vi "Termo_1.5__.vi"() -> ()   [LabVIEW 2015]
doc: "Программа мониторинга температуры"
uses:
  <vilib>/Utility/error.llb/DialogType.ctl
panel:
  in  "GraphLookB":bool
  out "Сутки":string
  out "счетчик":u32=4001
  in  "T min":u16=3 min=1 max=350
  in  "T max":u16=300 min=2 max=500
  in  "xScale -":bool
  in  "xScale +":bool
  out "мин.":string="20"
  out "TCP error source":string
  in  "порт":u16=4001
  in  "IP-адрес":string="10.10.10.2"
  out "Связь с прибором":bool
  in  "Disconnect":bool caption="Disconn"
  in  "Connect":bool
  out "3":bool
  out "1":bool
  out "2":bool
  out "Спаи":dbl format="%#_3g"
  out "K\n          Ом":dbl format="%#_5f"
  out "K\n          Ом 8":dbl format="%#_5f"
  out "K\n          Ом 7":dbl format="%#_5f"
  out "K\n          Ом 6":dbl format="%#_5f"
  out "Сол.":dbl format="%#_3g"
  out "Стр.":dbl format="%#_3g"
  out "Пер.":dbl format="%#_3g"
  out "4 2":bool
  in  "Запись в файл":bool
  out "сек.":string="0"
  out "часы":string="0"
  in  "Добавить время":dbl(ring)=300.0 items=["1 сек."=1.0, "10 сек."=10.0, "1 мин."=60.0, "5 мин."=300.0, "10 мин."=600.0, "1 час"=3600.0, ""=0.0]
  in  "stop":bool
  out "con err":bool caption="Connect"
  out "Graphs":dynamicdata(graph)
  out "read_error_indicator":bool
  out "refnum out":refnum<file>
  in  "flag1":bool caption="Disconn"
  out "x+1":dbl
  out "connection ID":refnum<k5>
  out "Расположение файла":path
  # "R [Ом]"
  # "T [K] [K]"
  # "Стр."
  # "Спаи"
  # "Пер."
  # "Сол."
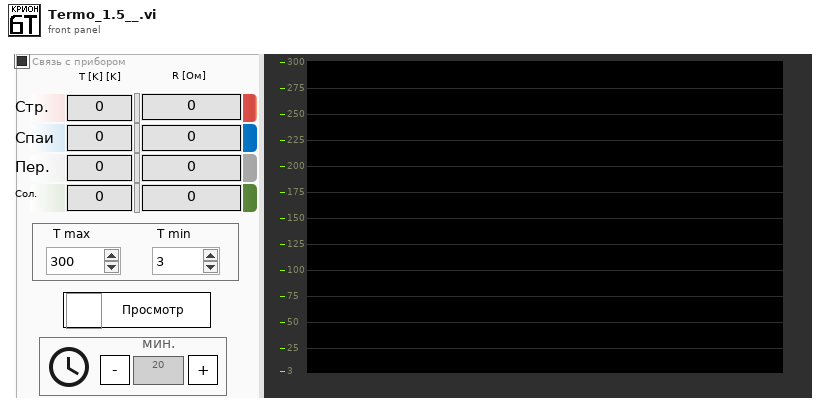
[diagram p1: front panel]
types:
  T1 = typedef "LVDateTimeRec.ctl" = cluster{"fractional second":dbl, "second":i32, "minute":i32, "hour":i32, "day of month":i32, "month":i32, "year":i32, "day of week":i32, "day of year":i32, "DST":i32}
  T2 = enum16{"Standard", "Buffered", "CRLF", "Immediate"}
  T3 = cluster{"y":ext, "y":ext, "y":ext, "y":ext, "y":ext, "y":ext, "y":ext}
  T4 = typedef "DialogType.ctl" = u16
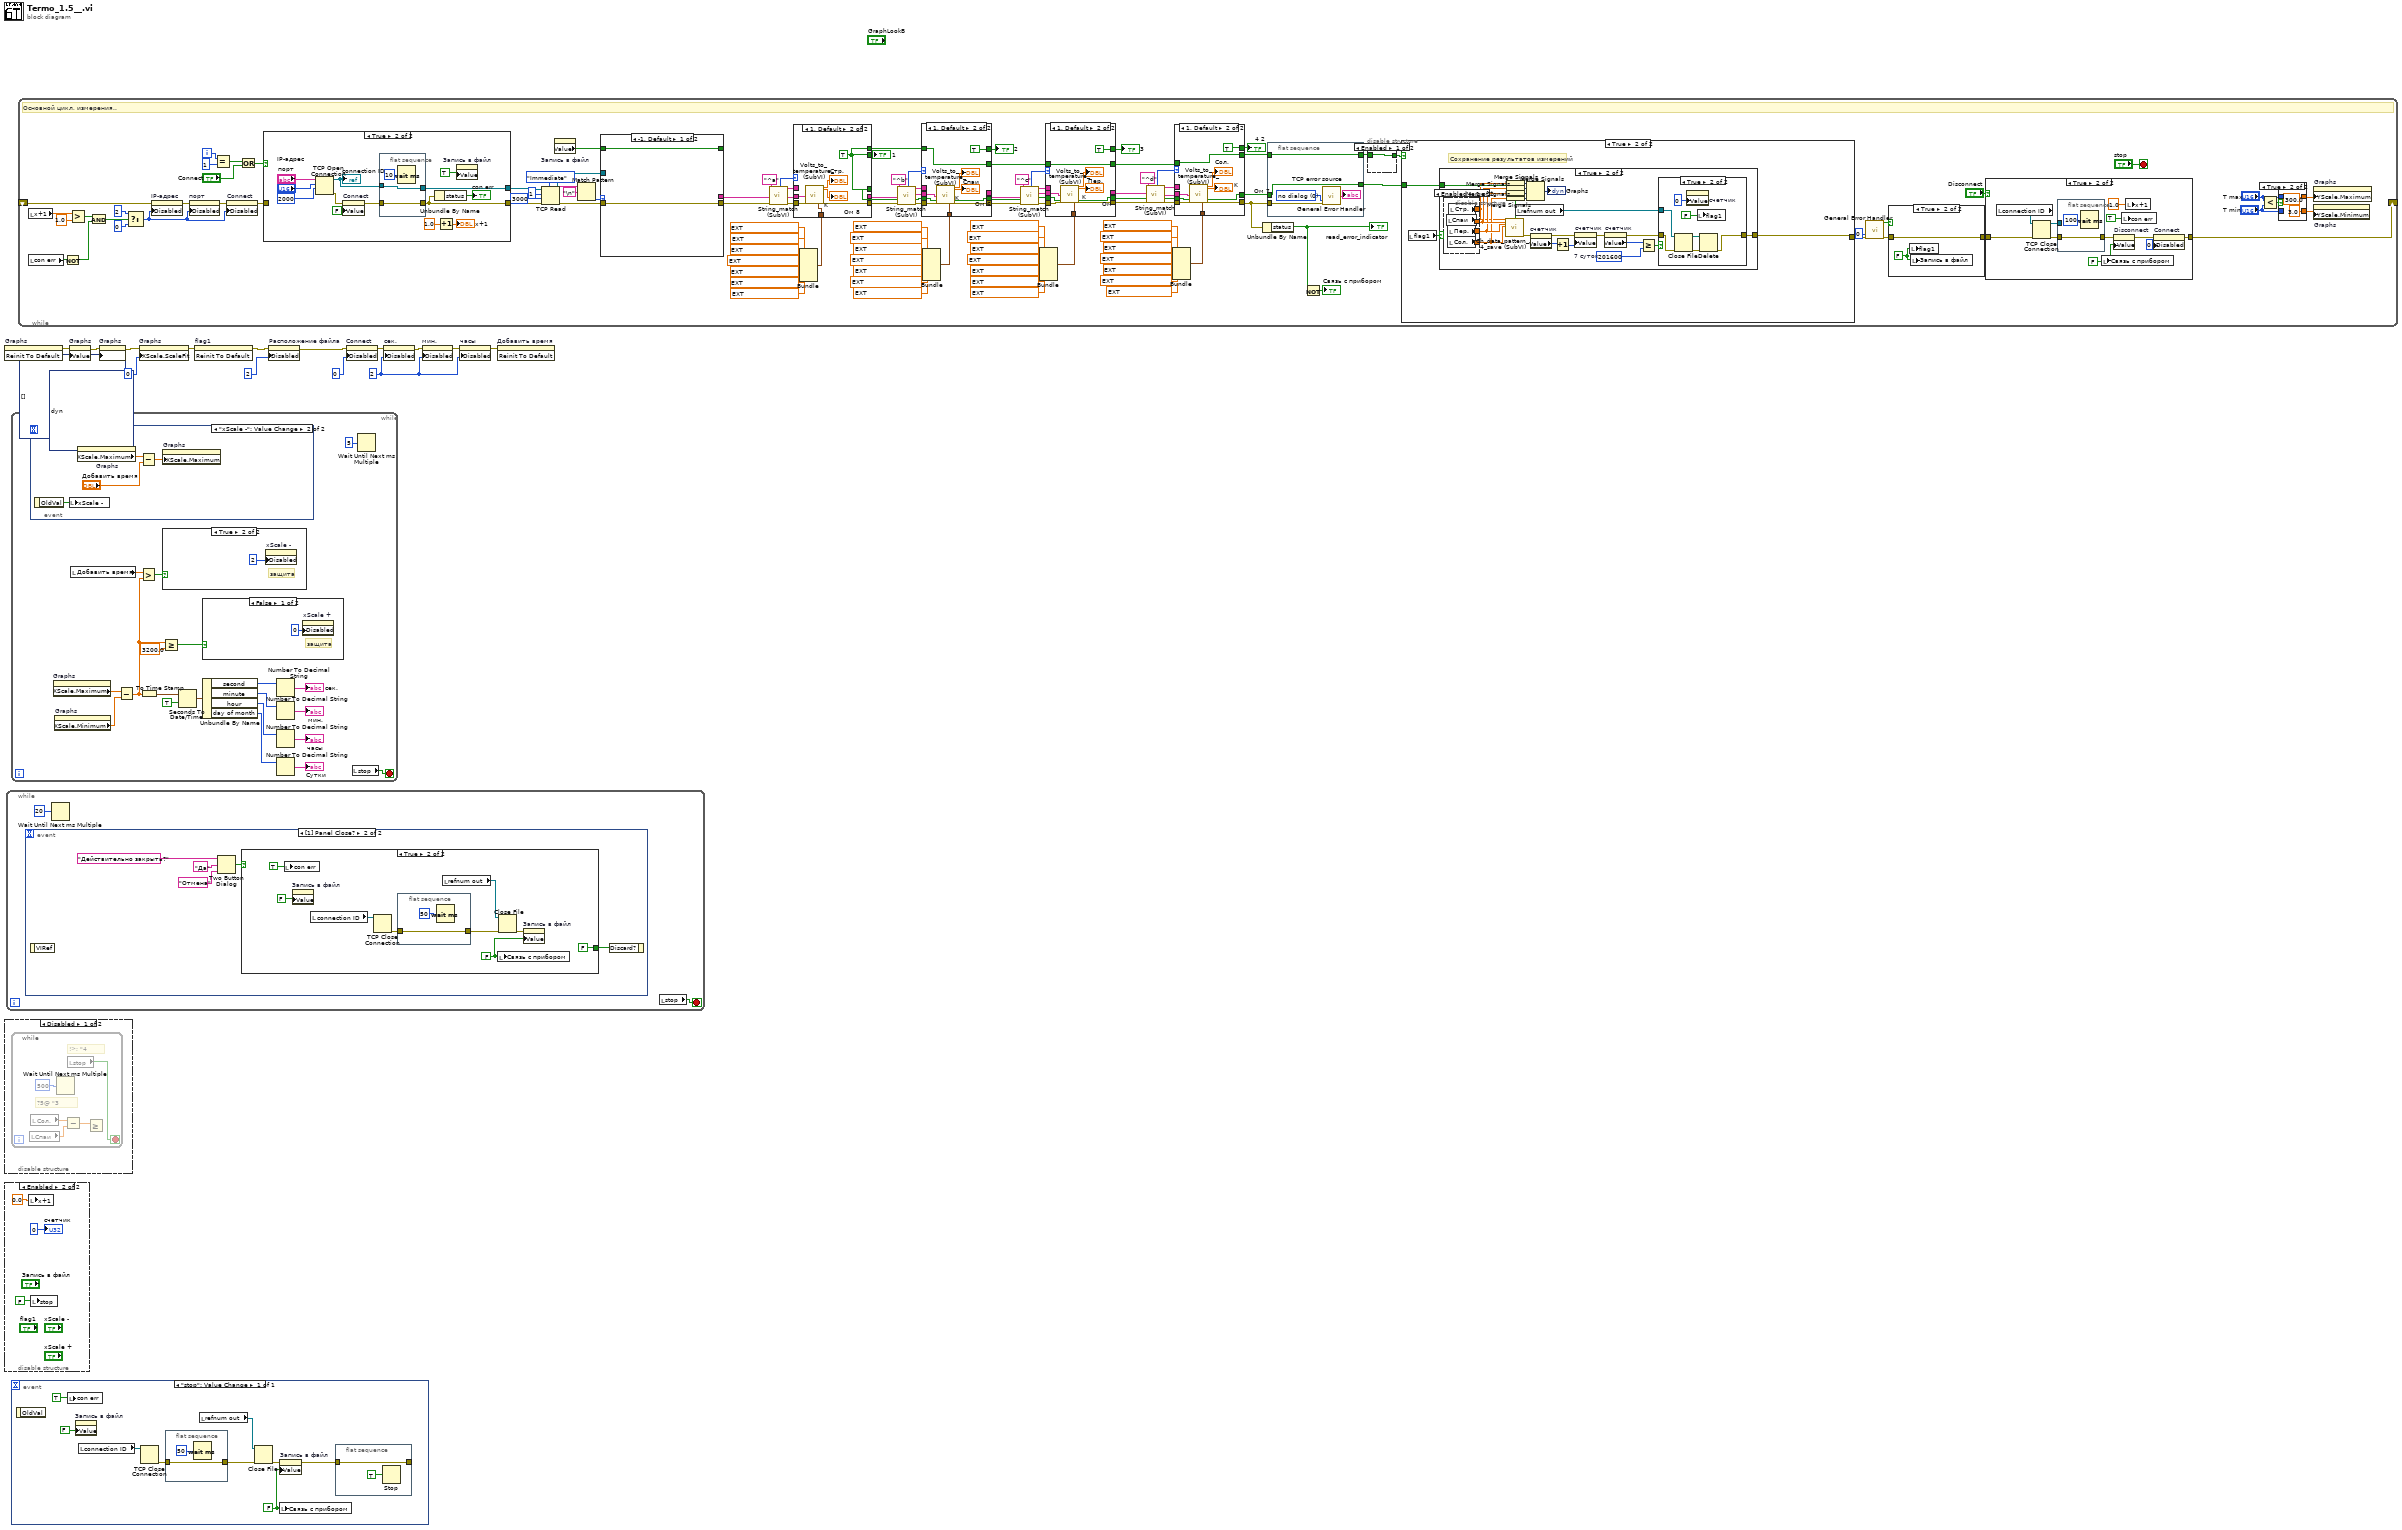
[diagram p0: block diagram]
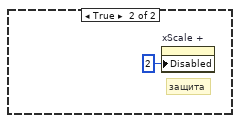
[diagram p2: hidden frame]
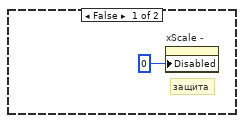
[diagram p3: hidden frame]
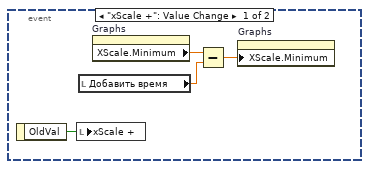
[diagram p4: hidden frame]
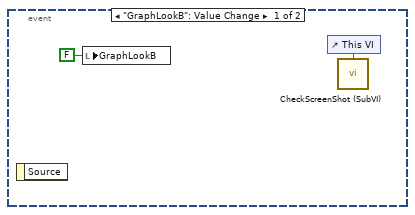
[diagram p7: hidden frame]
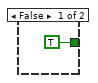
[diagram p8: hidden frame]
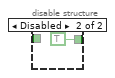
[diagram p9: hidden frame]
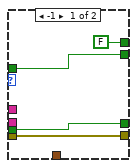
[diagram p11: hidden frame]
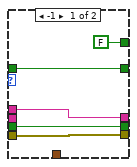
[diagram p12: hidden frame]
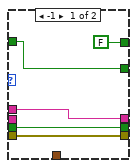
[diagram p13: hidden frame]
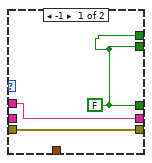
[diagram p14: hidden frame]
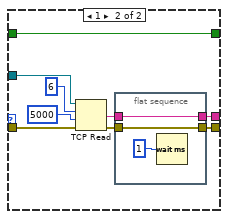
[diagram p15: hidden frame]
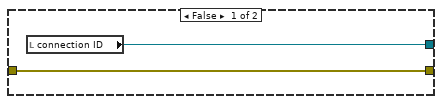
[diagram p16: hidden frame]
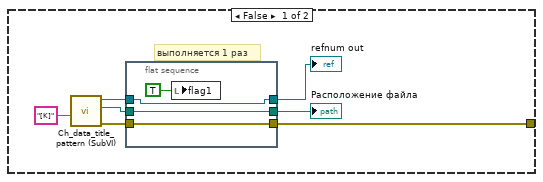
[diagram p19: hidden frame]
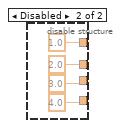
[diagram p20: hidden frame]
diagram:
  w15 = u8 2 ("Disabled")
  n1 = invoke on="Graphs" class="WFChart (strict)" method="Reinit To Default"() -> (error out=w7:errorcluster)  [unwired: 3 in, 2 out]
  n2 = disable-structure shown="Disabled" {
    frame Disabled {
      n3 = while {
        stop <- w23 stop-if-true
        # "!>; \"4"
        # "?5@ \"3"
        n4 = local read "Спаи"() -> (w19:dbl)
        n5 = local read "Сол."() -> (w20:dbl)
        n6 = Wait Until Next ms Multiple(millisecond multiple=u32 500) -> ()  [unwired: 1 out]
        n7 = Subtract(x=w20, y=w19) -> (x-y=w17:dbl)
        n8 = local read "stop"() -> (w23:bool)
        n9 = Greater Or Equal?(x=w17) -> (y=w18:dbl, x >= y?=w21:bool)
      }
    }
    frame Enabled {
    }
  }
  n10 = disable-structure shown="Enabled" {
    frame Disabled {
    }
    frame Enabled {
      n11 = local write "x+1"(0.0 ("x+1")) -> ()
      n12 = local write "stop"(FALSE ("Boolean")) -> ()
      "счетчик" <- u32 0 ("счетчик")
    }
  }
  n13 = while {
    stop <- w27 stop-if-true
    n14 = event shown="[1] Panel Close?" {
      selector: _ -> [_ _]
      dyn-events: _ -> [_ _]
      timeout: _ -> [_ _]
      event "GraphLookB": Value Change {
        n15 = event-data() -> ()  [unwired: 2 out]
        n16 = local write "GraphLookB"(FALSE ("Снимок")) -> ()
        n17 = control-ref of="This VI"() -> (w29:refnum<vi>)
        n18 = call "CheckScreenShot (SubVI).vi"("VI reference"=w29) -> ()  [unwired: 15 in]
      }
      event Panel Close? {
        n19 = event-data() -> ()  [unwired: 2 out]
        n20 = Two Button Dialog(message="Действительно закрыть?", 1:"Отмена" ("T button name (\"OK\")"), 2:"Да" ("T button name (\"OK\")")) -> (T button?=w35:bool)
        n21 = case shown="True" w35 {
          tunnel: [TRUE ("Discard?") FALSE ("Discard?")] -> w31
          frame False {
          }
          frame True {
            w42 = FALSE ("Запись в файл")
            n22 = local write "con err"(TRUE ("Tool Bar:Visible")) -> ()
            n23 = property on="Запись в файл" class="Bool (strict)"("Value"=FALSE ("Запись в файл")) -> ()  [unwired: 2 in, 2 out]
            n24 = local read "connection ID"() -> (w38:refnum<k5>)
            n25 = TCP Close Connection(connection ID=w38) -> (error out=w45:errorcluster)  [unwired: 1 in, 2 out]
            n26 = flat-sequence {
              tunnel: [w46] -> w44
              tunnel: w45 -> [w46]
              frame #0 {
                n27 = Wait (ms)(milliseconds to wait=u32 50) -> ()  [unwired: 1 out]
              }
            }
            n28 = local read "refnum out"() -> (w40:refnum<file>)
            n29 = local write "Связь с прибором"(w42) -> ()
            n30 = Close File(refnum=w40, error in=w44) -> (error out=w39:errorcluster)  [unwired: 1 out]
            n31 = property on="Запись в файл" class="Bool (strict)"(error in=w39, "Value"=w42) -> ()  [unwired: 1 in, 2 out]
          }
        }
        n32 = event-data("Discard?"=w31) -> ()  [unwired: 1 in, 1 out]
      }
    }
    n33 = Wait Until Next ms Multiple(millisecond multiple=u32 20) -> ()  [unwired: 1 out]
    n34 = local read "stop"() -> (w27:bool)
  }
  n35 = while {
    stop <- w67 stop-if-true
    n36 = event shown="[1] \"xScale -\": Value Change" {
      selector: _ -> [_ _]
      dyn-events: _ -> [_ _]
      timeout: _ -> [_ _]
      event "xScale +": Value Change {
        n37 = event-data() -> ("OldVal"=w72:bool)  [unwired: 1 in]
        n38 = local write "xScale +"(w72) -> ()
        n39 = local read "Добавить время"() -> (w75:dbl)
        n40 = property on="Graphs" class="WFChart (strict)"() -> ("XScale.Minimum"=w74:dbl)  [unwired: 2 in, 2 out]
        n41 = Subtract(x=w74, y=w75) -> (x-y=w73:dbl)
        n42 = property on="Graphs" class="WFChart (strict)"("XScale.Minimum"=w73) -> ()  [unwired: 2 in, 2 out]
      }
      event "xScale -": Value Change {
        n43 = event-data() -> ("OldVal"=w76:bool)  [unwired: 1 in]
        n44 = local write "xScale -"(w76) -> ()
        n45 = property on="Graphs" class="WFChart (strict)"() -> ("XScale.Maximum"=w78:dbl)  [unwired: 2 in, 2 out]
        n46 = Subtract(x=w78, y="Добавить время") -> (x-y=w77:dbl)
        n47 = property on="Graphs" class="WFChart (strict)"("XScale.Maximum"=w77) -> ()  [unwired: 2 in, 2 out]
      }
    }
    n48 = property on="Graphs" class="WFChart (strict)"() -> ("XScale.Maximum"=w66:dbl)  [unwired: 2 in, 2 out]
    n49 = property on="Graphs" class="WFChart (strict)"() -> ("XScale.Minimum"=w65:dbl)  [unwired: 2 in, 2 out]
    n50 = local read "Добавить время"() -> (w63:dbl)
    n51 = Subtract(x=w66, y=w65) -> (x-y=w51:dbl)
    n52 = Greater?(x=w63, y=w51) -> (0:w64:bool)
    n53 = To Time Stamp(1:w51) -> (0:w61:timestamp)
    n54 = Greater Or Equal?(x=w51, y=3200.0) -> (x >= y?=w49:bool)
    n55 = case shown="True" w64 {
      frame False {
        # "защита"
        n56 = property on="xScale -" class="Bool (strict)"("Disabled"=u8 0) -> ()  [unwired: 2 in, 2 out]
      }
      frame True {
        # "защита"
        n57 = property on="xScale -" class="Bool (strict)"("Disabled"=u8 2) -> ()  [unwired: 2 in, 2 out]
      }
    }
    n58 = Seconds To Date/Time(time stamp (now)=w61, to UTC (F)=TRUE) -> (date time rec=w60:T1)
    n59 = case shown="False" w49 {
      frame False {
        # "защита"
        n60 = property on="xScale +" class="Bool (strict)"("Disabled"=u8 0) -> ()  [unwired: 2 in, 2 out]
      }
      frame True {
        # "защита"
        n61 = property on="xScale +" class="Bool (strict)"("Disabled"=u8 2) -> ()  [unwired: 2 in, 2 out]
      }
    }
    n62 = Unbundle By Name(w60) -> ("second"=w59:i32, "minute"=w58:i32, "hour"=w57:i32, "day of month"=w56:i32)
    n63 = Number To Decimal String(number=w59) -> (decimal integer string=→"сек.":string)  [unwired: 1 out]
    n64 = Number To Decimal String(number=w58) -> (decimal integer string=→"мин.":string)  [unwired: 1 out]
    n65 = Number To Decimal String(number=w57) -> (decimal integer string=→"часы":string)  [unwired: 1 out]
    n66 = Number To Decimal String(number=w56) -> (decimal integer string=→"Сутки":string)  [unwired: 1 out]
    n67 = local read "stop"() -> (w67:bool)
    n68 = Wait Until Next ms Multiple(millisecond multiple=u32 5) -> ()  [unwired: 1 out]
  }
  n69 = event shown="[0] \"stop\": Value Change" {
    selector: _ -> [_]
    dyn-events: _ -> [_]
    timeout: _ -> [_]
    event "stop": Value Change {
      w85 = FALSE ("Запись в файл")
      n70 = event-data() -> ()  [unwired: 1 in, 1 out]
      n71 = local write "con err"(TRUE ("Tool Bar:Visible")) -> ()
      n72 = property on="Запись в файл" class="Bool (strict)"("Value"=FALSE ("Запись в файл")) -> ()  [unwired: 2 in, 2 out]
      n73 = local read "connection ID"() -> (w81:refnum<k5>)
      n74 = TCP Close Connection(connection ID=w81) -> (error out=w88:errorcluster)  [unwired: 1 in, 2 out]
      n75 = flat-sequence {
        tunnel: [w91] -> w87
        tunnel: w88 -> [w91]
        frame #0 {
          n76 = Wait (ms)(milliseconds to wait=u32 50) -> ()  [unwired: 1 out]
        }
      }
      n77 = local read "refnum out"() -> (w83:refnum<file>)
      n78 = Close File(refnum=w83, error in=w87) -> (error out=w82:errorcluster)  [unwired: 1 out]
      n79 = property on="Запись в файл" class="Bool (strict)"(error in=w82, "Value"=w85) -> (error out=w80:errorcluster)  [unwired: 1 in, 1 out]
      n80 = local write "Связь с прибором"(w85) -> ()
      n81 = flat-sequence {
        tunnel: w80 -> [w90]
        tunnel: [w90] -> _
        frame #0 {
          n82 = Stop(stop? (T)=TRUE) -> ()
        }
      }
    }
  }
  n83 = while {
    shift-right: [w103] -> _
    shift-left: _ -> [w192]
    i -> [w178]
    stop <- "stop" stop-if-true
    # "Основной цикл, измерения.."
    n84 = local read "x+1"() -> (w214:dbl)
    n85 = local read "con err"() -> (w210:bool)
    n86 = Not(x=w210) -> (.not. x?=w209:bool)
    n87 = Greater?(x=w214, y=1.0) -> (0:w212:bool)
    n88 = And(x=w212, y=w209) -> (x .and. y?=w194:bool)
    n89 = Select(t=u8 2 ("Disabled"), s=w194, f=u8 0 ("Disabled")) -> (s? t:f=w138:u8)
    n90 = property on="IP-адрес" class="Str"(error in=w192, "Disabled"=w138) -> (error out=w193:errorcluster)  [unwired: 1 in, 1 out]
    n91 = property on="порт" class="DigNum (strict)"(error in=w193, "Disabled"=w138) -> (error out=w191:errorcluster)  [unwired: 1 in, 1 out]
    n92 = Equal?(x=w178, y=1) -> (x = y?=w184:bool)
    n93 = property on="Connect" class="Bool (strict)"(error in=w191, "Disabled"=w138) -> (error out=w176:errorcluster)  [unwired: 1 in, 1 out]
    n94 = Or(x=w184, y="Connect") -> (x .or. y?=w186:bool)
    n95 = case shown="True" w186 {
      tunnel: [w291 w293] -> w188
      tunnel: [w290 w295] -> w187
      tunnel: w176 -> [w291 _]
      frame False {
        n96 = local read "connection ID"() -> (w290:refnum<k5>)
      }
      frame True {
        n97 = TCP Open Connection(address="IP-адрес", remote port or service name="порт", timeout ms (60000)=2000) -> (connection ID=w296:refnum<k5>, error out=w298:errorcluster)  [unwired: 1 in, 1 out]
        "connection ID" <- w296
        n98 = property on="Connect" class="Bool (strict)"(error in=w298, "Value"=FALSE ("Connect")) -> (error out=w297:errorcluster)  [unwired: 1 in, 1 out]
        n99 = flat-sequence {
          tunnel: w297 -> [w306]
          tunnel: [w306] -> w293
          tunnel: w296 -> [w305]
          tunnel: [w305] -> w295
          frame #0 {
            n100 = Wait (ms)(milliseconds to wait=u32 10) -> ()  [unwired: 1 out]
          }
        }
        n101 = Unbundle By Name(w293) -> ("status"=→"con err":bool)
        n102 = Increment(x=1.0) -> (x+1=→"x+1":dbl)
        n103 = property on="Запись в файл" class="Bool (strict)"("Value"=TRUE ("Запись в файл")) -> ()  [unwired: 2 in, 2 out]
      }
    }
    n104 = TCP Read(connection ID=w187, bytes to read=1, error in (no error)=w188, 7:T2."Immediate" ("mode (standard)"), 9:3000 ("timeout ms (25000)")) -> (connection ID out=w189:refnum<k5>, data out=w190:string, error out=w174:errorcluster)
    n105 = property on="Запись в файл" class="Bool (strict)"() -> ("Value"=w105:bool)  [unwired: 2 in, 2 out]
    n106 = Match Pattern(string=w190, regular expression="\n") -> (offset past match=w183:i32)  [unwired: 4 out]
    n107 = case shown="-1, Default" w183 {
      tunnel: [w277 w286] -> w171
      tunnel: [_ w285] -> w175
      tunnel: w189 -> [_ w284]
      tunnel: w174 -> [w277 w283]
      tunnel: [w276 w278] -> _
      tunnel: w105 -> [w276 w278]
      frame -1, Default {
      }
      frame 1 {
        n108 = TCP Read(connection ID=w284, bytes to read=6, error in (no error)=w283, 9:5000 ("timeout ms (25000)")) -> (data out=w279:string, error out=w280:errorcluster)  [unwired: 2 out]
        n109 = flat-sequence {
          tunnel: w280 -> [w288]
          tunnel: [w288] -> w286
          tunnel: [w287] -> w285
          tunnel: w279 -> [w287]
          frame #0 {
            n110 = Wait (ms)(milliseconds to wait=u32 1) -> ()  [unwired: 1 out]
          }
        }
      }
    }
    n111 = call "String_match (SubVI).vi"("channel id"="^a" ("regular expression"), "input string"=w175, "error in"=w171) -> ("match ?"=w168:i32, "output string"=w165:string, "match substring"=w166:string, "error out"=w167:errorcluster)  [unwired: 12 in, 1 out]
    n112 = Bundle("y"=ext 12.1972840491798706, "y"=ext -103.27107382635586, "y"=ext 397.925821471959352, "y"=ext -567.703864333219826, "y"=ext 208.59269304759800399, "y"=ext 315.492219684645534, "y"=ext -92.57400480215438) -> (w130:T3)  [unwired: 1 in]
    n113 = case shown="1, Default" w168 {
      tunnel: [w268 w275] -> w142
      tunnel: [w266 w269] -> w170
      tunnel: [w266 w269] -> w207
      tunnel: w167 -> [w268 w274]
      tunnel: w166 -> [_ w270]
      tunnel: [w267 _] -> w206
      tunnel: w165 -> [w267 _]
      tunnel: [w266 w269] -> w201
      tunnel: w130 -> [_ w271]
      frame -1 {
        w266 = FALSE ("1")
      }
      frame 1, Default {
        w269 = TRUE ("1")
        n114 = call "Volts_to_temperature_(SubVI).vi"("ch_data_string"=w270, "error in"=w274, "koeff. cluster"=w271) -> ("T solvation"=→"Стр.":dbl, "meas_voltage"=→"K\n          Ом 8":dbl, "error out"=w275:errorcluster)  [unwired: 21 in, 1 out]
      }
    }
    "1" <- w170
    n115 = call "String_match (SubVI).vi"("channel id"="^b" ("regular expression"), "input string"=w206, "Boolean in"=w207, "error in"=w142) -> ("match ?"=w162:i32, "output string"=w158:string, "match substring"=w159:string, "Boolean out"=w161:bool, "error out"=w160:errorcluster)  [unwired: 11 in]
    n116 = Bundle("y"=ext 3.06244888759101741, "y"=ext -30.3586341044865549, "y"=ext 241.908977336715907, "y"=ext -649.75628893822431598, "y"=ext 955.307573420926928, "y"=ext -485.428257496096194, "y"=ext 136.248866791371256) -> (w122:T3)  [unwired: 1 in]
    n117 = case shown="1, Default" w162 {
      tunnel: [w254 w265] -> w141
      tunnel: [FALSE ("1") TRUE ("1")] -> w164
      tunnel: w161 -> [w253 w263]
      tunnel: w160 -> [w254 w262]
      tunnel: w159 -> [_ w261]
      tunnel: [w253 w260] -> w205
      tunnel: w158 -> [w252 _]
      tunnel: [w252 _] -> w204
      tunnel: w201 -> [w251 w259]
      tunnel: [w251 w259] -> w200
      tunnel: w122 -> [_ w256]
      frame -1 {
      }
      frame 1, Default {
        n118 = call "Volts_to_temperature_(SubVI).vi"("ch_data_string"=w261, "Boolean in"=w263, "error in"=w262, "koeff. cluster"=w256) -> ("T solvation"=→"Спаи":dbl, "meas_voltage"=→"K\n          Ом 6":dbl, "Boolean out"=w260:bool, "error out"=w265:errorcluster)  [unwired: 20 in]
      }
    }
    "2" <- w164
    n119 = call "String_match (SubVI).vi"("channel id"="^c" ("regular expression"), "input string"=w204, "Boolean in"=w205, "error in"=w141) -> ("match ?"=w153:i32, "output string"=w152:string, "match substring"=w151:string, "Boolean out"=w155:bool, "error out"=w156:errorcluster)  [unwired: 11 in]
    n120 = Bundle("y"=ext 17.256671486888080801, "y"=ext -215.322746395599097, "y"=ext 1219.40785944648087, "y"=ext -3277.70955596119165, "y"=ext 4778.55193661898375, "y"=ext -3251.6292140185833, "y"=ext 954.333331361413) -> (w114:T3)  [unwired: 1 in]
    n121 = case shown="1, Default" w153 {
      tunnel: w156 -> [w239 w250]
      tunnel: [w239 w249] -> w140
      tunnel: [w238 _] -> w203
      tunnel: [FALSE ("1") TRUE ("1")] -> w157
      tunnel: w155 -> [w237 w247]
      tunnel: w152 -> [w238 _]
      tunnel: w151 -> [_ w246]
      tunnel: [w237 w245] -> w202
      tunnel: w200 -> [w236 w244]
      tunnel: [w236 w244] -> w199
      tunnel: w114 -> [_ w241]
      frame -1 {
      }
      frame 1, Default {
        n122 = call "Volts_to_temperature_(SubVI).vi"("ch_data_string"=w246, "Boolean in"=w247, "error in"=w250, "koeff. cluster"=w241) -> ("T solvation"=→"Пер.":dbl, "meas_voltage"=→"K\n          Ом":dbl, "Boolean out"=w245:bool, "error out"=w249:errorcluster)  [unwired: 20 in]
      }
    }
    "3" <- w157
    n123 = call "String_match (SubVI).vi"("channel id"="^d" ("regular expression"), "input string"=w203, "Boolean in"=w202, "error in"=w140) -> ("match ?"=w148:i32, "output string"=w145:string, "match substring"=w146:string, "Boolean out"=w147:bool, "error out"=w149:errorcluster)  [unwired: 11 in]
    n124 = Bundle("y"=ext 4.0050674039521255, "y"=ext -55.2455571058671922, "y"=ext 448.087557092308998, "y"=ext -1390.99036489240825, "y"=ext 2271.71780132129788, "y"=ext -1387.04864621348679, "y"=ext 500.36806705314666) -> (w106:T3)  [unwired: 1 in]
    n125 = case shown="1, Default" w148 {
      tunnel: w149 -> [w224 w235]
      tunnel: [w224 w234] -> w139
      tunnel: [FALSE ("1") TRUE ("1")] -> w104
      tunnel: w147 -> [w223 w230]
      tunnel: w146 -> [_ w229]
      tunnel: w145 -> [_ _]
      tunnel: [w223 w228] -> w143
      tunnel: w199 -> [w222 w227]
      tunnel: [w222 w227] -> w144
      tunnel: w106 -> [_ w226]
      frame -1 {
      }
      frame 1, Default {
        n126 = call "Volts_to_temperature_(SubVI).vi"("ch_data_string"=w229, "Boolean in"=w230, "error in"=w235, "koeff. cluster"=w226) -> ("T solvation"=→"Сол.":dbl, "meas_voltage"=→"K\n          Ом 7":dbl, "Boolean out"=w228:bool, "error out"=w234:errorcluster)  [unwired: 20 in]
      }
    }
    "4 2" <- w104
    n127 = Unbundle By Name(w139) -> ("status"=w95:bool)
    "read_error_indicator" <- w95
    n128 = flat-sequence {
      tunnel: w139 -> [w311]
      tunnel: w144 -> [w309]
      tunnel: [w309] -> w93
      tunnel: w143 -> [w308]
      tunnel: [w308] -> w198
      frame #0 {
        w312 = T4 0 items=["no dialog", "OK message", "continue or stop message", "OK message + warnings", "continue/stop + warnings"] ("type of dialog (OK msg:1)")
        n129 = call <vilib>:"General Error Handler.vi"("type of dialog (OK msg:1)"=w312, "error in (no error)"=w311) -> ("source out"=→"TCP error source":string)  [unwired: 1 in, 12 out]
      }
    }
    n130 = Not(x=w95) -> (.not. x?=→"Связь с прибором":bool)
    n131 = disable-structure shown="Enabled" {
      disable-tunnel: [w216 TRUE ("1")] -> w94
      disable-tunnel: w93 -> [w216 _]
      frame Enabled {
      }
      frame Disabled {
      }
    }
    n132 = case shown="True" w94 {
      tunnel: [_ w317] -> w211
      tunnel: w198 -> [_ w316]
      frame False {
        # "Сохранение результатов измерений"
      }
      frame True {
        # "Сохранение результатов измерений"
        n133 = local read "flag1"() -> (w318:bool)
        n134 = case shown="True" w318 {
          tunnel: [w324 w340] -> w317
          tunnel: w316 -> [_ w350]
          frame False {
            # "выполняется 1 раз"
            n135 = call "Ch_data_title_pattern (SubVI).vi"("Единица измерений"="[K]") -> ("error out"=w325:errorcluster, "Path"=w321:path, "Byte Stream File out"=w320:refnum<file>)  [unwired: 8 in]
            n136 = flat-sequence {
              tunnel: w325 -> [w328]
              tunnel: [w328] -> w324
              tunnel: [w327] -> w322
              tunnel: w321 -> [w327]
              tunnel: w320 -> [w326]
              tunnel: [w326] -> w319
              frame #0 {
                n137 = local write "flag1"(TRUE ("flag1")) -> ()
              }
            }
            "Расположение файла" <- w322
            "refnum out" <- w319
          }
          frame True {
            w343 = u32 201600  # 7 суток
            n138 = disable-structure shown="Enabled" {
              disable-tunnel: [w354 2.0 ("2")] -> w334
              disable-tunnel: [w353 3.0 ("3")] -> w333
              disable-tunnel: [w352 4.0 ("4")] -> w332
              disable-tunnel: [w351 1.0 ("1")] -> w330
              frame Enabled {
                n139 = local read "Спаи"() -> (w354:dbl)
                n140 = local read "Пер."() -> (w353:dbl)
                n141 = local read "Сол."() -> (w352:dbl)
                n142 = local read "Стр."() -> (w351:dbl)
              }
              frame Disabled {
              }
            }
            n143 = Merge Signals(w330) -> (w337:dynamicdata)
            n144 = Merge Signals(w334) -> (w336:dynamicdata)
            n145 = Merge Signals(w333) -> (w335:dynamicdata)
            n146 = Merge Signals(w332) -> (w338:dynamicdata)
            n147 = local read "refnum out"() -> (w342:refnum<file>)
            n148 = call "Ch_data_pattern_4_save (SubVI).vi"("1"=w330, "2"=w334, "3"=w333, "4"=w332, "file"=w342, "Activate!"=w350) -> ("error out"=w346:errorcluster)  [unwired: 21 in]
            n149 = Merge Signals(w337, w336, w335, w338) -> (→"Graphs":dynamicdata)
            n150 = property on="счетчик" class="DigNum (strict)"(error in=w346) -> (error out=w349:errorcluster, "Value"=w347:u32)  [unwired: 1 in, 1 out]
            n151 = Increment(x=w347) -> (x+1=w348:u32)
            n152 = property on="счетчик" class="DigNum (strict)"(error in=w349, "Value"=w348) -> (error out=w345:errorcluster)  [unwired: 1 in, 1 out]
            n153 = property on="счетчик" class="DigNum (strict)"(error in=w345) -> (error out=w341:errorcluster, "Value"=w344:u32)  [unwired: 1 in, 1 out]
            n154 = Greater Or Equal?(x=w344, y=w343) -> (x >= y?=w339:bool)
            n155 = case shown="True" w339 {
              tunnel: w342 -> [_ w364]
              tunnel: w341 -> [w359 w363]
              tunnel: [w359 w362] -> w340
              frame False {
              }
              frame True {
                n156 = Close File(refnum=w364, error in=w363) -> (path=w365:path, error out=w366:errorcluster)
                n157 = property on="счетчик" class="DigNum (strict)"("Value"=u32 0 ("счетчик")) -> ()  [unwired: 2 in, 2 out]
                n158 = local write "flag1"(FALSE) -> ()
                n159 = Delete(path (use dialog)=w365, error in=w366) -> (error out=w362:errorcluster)  [unwired: 3 in, 2 out]
              }
            }
          }
        }
      }
    }
    n160 = call <vilib>:"General Error Handler.vi"("type of dialog (OK msg:1)"=u32 0 ("milliseconds to wait"), "error in (no error)"=w211) -> ("error?"=w173:bool, "error out"=w172:errorcluster)  [unwired: 1 in, 11 out]
    n161 = case shown="True" w173 {
      tunnel: w172 -> [w313 w314]
      tunnel: [w313 w314] -> w197
      frame False {
      }
      frame True {
        w315 = FALSE
        n162 = local write "flag1"(w315) -> ()
        n163 = local write "Запись в файл"(w315) -> ()
      }
    }
    n164 = case shown="True" "Disconnect" {
      tunnel: [w367 w369] -> w103
      tunnel: w197 -> [w367 w378]
      frame False {
      }
      frame True {
        w368 = FALSE ("Disconnect")
        n165 = local read "connection ID"() -> (w377:refnum<k5>)
        n166 = TCP Close Connection(connection ID=w377, error in (no error)=w378) -> (connection ID out=w372:refnum<k5>, error out=w371:errorcluster)  [unwired: 1 out]
        n167 = flat-sequence {
          tunnel: w372 -> [_]
          tunnel: w371 -> [w379]
          tunnel: [w379] -> w370
          frame #0 {
            n168 = Wait (ms)(milliseconds to wait=u32 100) -> ()  [unwired: 1 out]
          }
        }
        n169 = local write "Связь с прибором"(w368) -> ()
        n170 = property on="Disconnect" class="Bool (strict)"(error in=w370, "Value"=w368) -> (error out=w373:errorcluster)  [unwired: 1 in, 1 out]
        n171 = local write "con err"(TRUE ("con err")) -> ()
        n172 = local write "x+1"(1.0 ("1")) -> ()
        n173 = property on="Connect" class="Bool (strict)"(error in=w373, "Disabled"=u8 0) -> (error out=w369:errorcluster)  [unwired: 1 in, 1 out]
      }
    }
    n174 = Less?(x="T max", y="T min") -> (x < y?=w99:bool)
    n175 = case shown="True" w99 {
      tunnel: [w219 300.0 ("x+1")] -> w101
      tunnel: [w218 3.0 ("x+1")] -> w100
      tunnel: "T max" -> [w219 _]
      tunnel: "T min" -> [w218 _]
      frame False {
      }
      frame True {
      }
    }
    n176 = property on="Graphs" class="WFChart (strict)"("YScale.Maximum"=w101) -> ()  [unwired: 2 in, 2 out]
    n177 = property on="Graphs" class="WFChart (strict)"("YScale.Minimum"=w100) -> ()  [unwired: 2 in, 2 out]
  }
  n178 = property on="Graphs" class="WFChart (strict)"(error in=w7, "Value"=dynamicdata [{"t0"=timestamp(3465273261.7246556 s since 1904-01-01), "dt"=1.0, "Y"=[0.1931097262457384]}, {"t0"=timestamp(3465273261.7246556 s since 1904-01-01), "dt"=1.0, "Y"=[0.3594116459482981]}, {"t0"=timestamp(3465273261.7246556 s since 1904-01-01), "dt"=1.0, "Y"=[0.8898205452798131]}, {"t0"=timestamp(3465273261.7246556 s since 1904-01-01), "dt"=1.0, "Y"=[0.747699236883661]}] ("Graphs")) -> (error out=w9:errorcluster)  [unwired: 1 in, 1 out]
  n179 = property on="Graphs" class="WFChart (strict)"(error in=w9, "History Data"=dynamicdata[] []) -> (error out=w3:errorcluster)  [unwired: 1 in, 1 out]
  n180 = property on="Graphs" class="WFChart (strict)"(error in=w3, "XScale.ScaleFit"=u8 0 ("Y Scale.Scale Fit")) -> (error out=w2:errorcluster)  [unwired: 1 in, 1 out]
  n181 = invoke on="flag1" class="Bool (strict)" method="Reinit To Default"(error in=w2) -> (error out=w8:errorcluster)  [unwired: 2 in, 2 out]
  n182 = property on="Расположение файла" class="Path"(error in=w8, "Disabled"=u8 2) -> (error out=w1:errorcluster)  [unwired: 1 in, 1 out]
  n183 = property on="Connect" class="Bool (strict)"(error in=w1, "Disabled"=u8 0) -> (error out=w5:errorcluster)  [unwired: 1 in, 1 out]
  n184 = property on="сек." class="Str"(error in=w5, "Disabled"=w15) -> (error out=w12:errorcluster)  [unwired: 1 in, 1 out]
  n185 = property on="мин." class="Str"(error in=w12, "Disabled"=w15) -> (error out=w11:errorcluster)  [unwired: 1 in, 1 out]
  n186 = property on="часы" class="Str"(error in=w11, "Disabled"=w15) -> (error out=w10:errorcluster)  [unwired: 1 in, 1 out]
  n187 = invoke on="Добавить время" class="Ring (strict)" method="Reinit To Default"(error in=w10) -> ()  [unwired: 2 in, 3 out]
